vi "DB-通用exe查询模块.vi"(8 "error in (no error)":errorcluster, 9 "解析模式":enum16{"仅数值", "仅字符串", "数值与字符串"}(ring), 10 "SQL query":string, 11 "数据库连接引用":T1) -> (0 "error out":errorcluster, 1 "字符串数据":string[][](array[string]), 2 "数值数据":dbl[][](array[numeric]), 3 "数据库连接引用out":T1)   [LabVIEW 2013, in "数据库操作.lvclass"]
uses:
  <vilib>/addons/database/Connection.llb/Conn ObjectReference.ctl
  <vilib>/addons/database/Connection.llb/Conn Execute.vi
  <vilib>/addons/database/Recordset.llb/Rec Fetch Recordset Data (R).vi
  <vilib>/addons/database/_DB Variant To Data/Database Variant To Data.xnode
  <vilib>/addons/database/NI_Database_API.lvlib
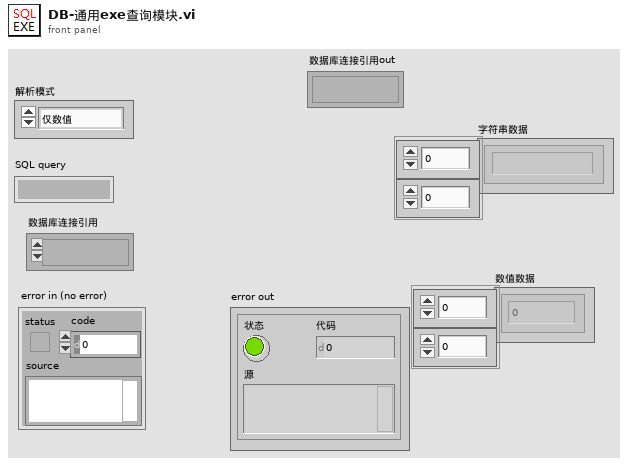
[diagram p1: front panel]
types:
  T1 = typedef "NI_Database_API.lvlib/Conn ObjectReference.ctl" = refnum<k1>
  T2 = typedef "NI_Database_API.lvlib/Rec ObjectReference.ctl" = refnum<k1>
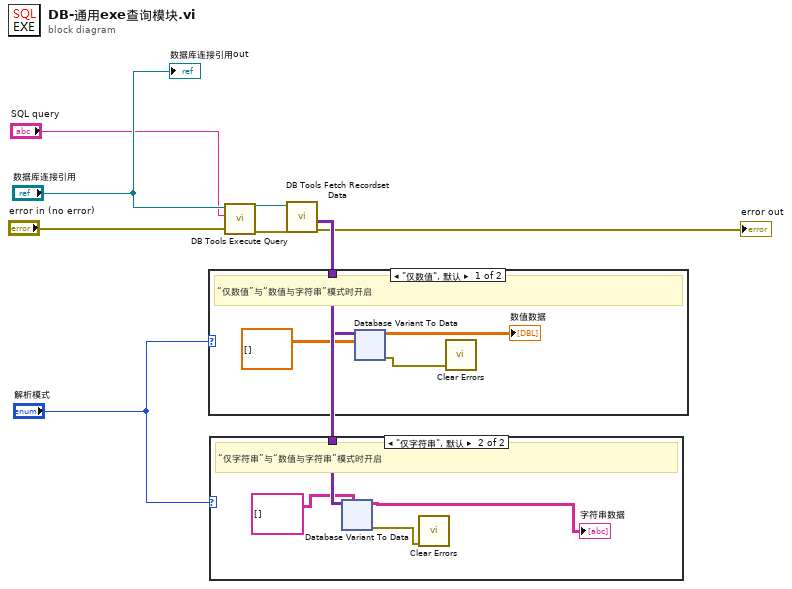
[diagram p0: block diagram]
diagram:
  n1 = call-poly <vilib>:"DB Tools Execute Query.vi"("error in (no error)"="error in (no error)", "SQL query"="SQL query", "connection reference"="数据库连接引用") -> ("error out"=w7:errorcluster, "recordset reference"=w6:T2)  [unwired: 5 in]
  n2 = call-poly <vilib>:"DB Tools Fetch Recordset Data.vi"("error in (no error)"=w7, "recordset reference"=w6) -> ("error out"=→"error out":errorcluster, "recordset data"=w3:variant[][])  [unwired: 3 in, 1 out]
  n3 = case shown="\"仅数值\", 默认" "解析模式" {
    tunnel: w3 -> [w11 _]
    frame "仅数值", Default {
      # "“仅数值”与“数值与字符串”模式时开启"
      n4 = xnode "Database Variant To Data"("database variant"=w11, "type"=dbl[][] []) -> ("data"=→"数值数据":dbl[][], "error out"=w9:errorcluster)  [unwired: 1 in]
      n5 = call <vilib>:"Clear Errors.vi"("error in (no error)"=w9) -> ()  [unwired: 6 in, 1 out]
    }
    frame "仅字符串" {
    }
  }
  n6 = case shown="\"仅字符串\", 默认" "解析模式" {
    tunnel: w3 -> [_ w60]
    frame "仅数值" {
    }
    frame "仅字符串", Default {
      # "“仅字符串”与“数值与字符串”模式时开启"
      n7 = xnode "Database Variant To Data"("database variant"=w60, "type"=string[][] []) -> ("data"=→"字符串数据":string[][], "error out"=w57:errorcluster)  [unwired: 1 in]
      n8 = call <vilib>:"Clear Errors.vi"("error in (no error)"=w57) -> ()  [unwired: 6 in, 1 out]
    }
  }
  "数据库连接引用out" <- "数据库连接引用"
